vi "XOR Tester.vi"() -> ()   [LabVIEW 2013, in "Super Simple Neural Network.lvlib"]
uses:
  Super Simple Neural Network.lvlib
  <vilib>/Math Plots/3D Math Plots/3D Surface/3D Surface XCtrl/3D Surface.xctl
  <vilib>/Math Plots/3D Math Plots/3D Surface/3D Surface Datatype/3D Surface Datatype.lvclass
  Types/Stop Settings.ctl
  Types/Error Evaluation.ctl
panel:
  out "Response Surface":refnum<class "3D Plot Datatype.lvclass">[](xcontrol)
  in  "1st Hidden Layer Neurons":i32=2
  out "Goal Reached":bool=TRUE
  out "Error Trend":dbl[](graph)=[1.2002969476479681, 1.2003117160068655, 1.1995748068252734, 1.1986266775824506, 1.1980759314790428, 1.1979331980453334, 1.1976182630837475, 1.1975531304739626, 1.1975550658555898, 1.1979172951382462, 1.1980082841901254, 1.1978288179593928, 1.1976548206695512, 1.1975294735041757, 1.1971542016928627, 1.1967580661942594, 1.196216870199815, 1.195587636803456, 1.1947866780682184, 1.1937807789025867, 1.1926114580938205, 1.1911927459665133, 1.189611032453872, 1.1879425541706663, 1.1845149684498697, 1.1790670045354323, 1.17271337283506, 1.1648553404478168, 1.154971369668143, 1.1429811791798623, 1.1413485366821972, 1.1363483063148954, 1.1285959137026458, 1.1183842954352032, 1.1000568961697912, 1.083998923386862, 1.0794867997140547, 1.0684617721747578, 1.0553434826869061, 1.0396958392495204, 1.02101123534143, 0.9870568895525247, 0.9538717523120656, 0.9292072809802745, 0.9277611383844048, 0.920217692956792, 0.9084926670755543, 0.8774111592803272, 0.8469460769163291, 0.8376337144337398, 0.8100956788583408, 0.7808588146654515, 0.7464611009002428, 0.7164446834205364, 0.6860931635965195, 0.6642874827461767, 0.6461698055293237, 0.6016389331387895, 0.5521940551327592, 0.4989840147890163, 0.46441855327952186, 0.41729315960747854, 0.3703383060113925, 0.3405465537992886, 0.3273094582704069, 0.3337348036757197, 0.33928987259102134, 0.3351085676703055, 0.33232405100150914, 0.3149530937747707, 0.29789405799141794, 0.28600474402962706, 0.28456326623217576, 0.2907819179767071, 0.2921232072153035, 0.2940047293155137, 0.2879779909912136, 0.28246444258404346, 0.2756352726767302, 0.26772935920574203, 0.25842195851389893, 0.2474992301012963, 0.2273583014029358, 0.2087320931456691, 0.18863310369744024, 0.1775969638076887, 0.1592192620834864, 0.1377098111297188, 0.11267838671254482, 0.08249869363894832]
  in  "Output Neurons/Outputs":i32=1
  in  "# Inputs":i32=2
  # "The succes rate for finding \na solution to the XOR \nproblem is smaller \nthan 100%. Sometimes you \nneed to re-run\nthe example multiple times.\n\nThe values of XOR are not 0\nand 1 to present the ability\nto scale inputs and outputs\ninside the API."
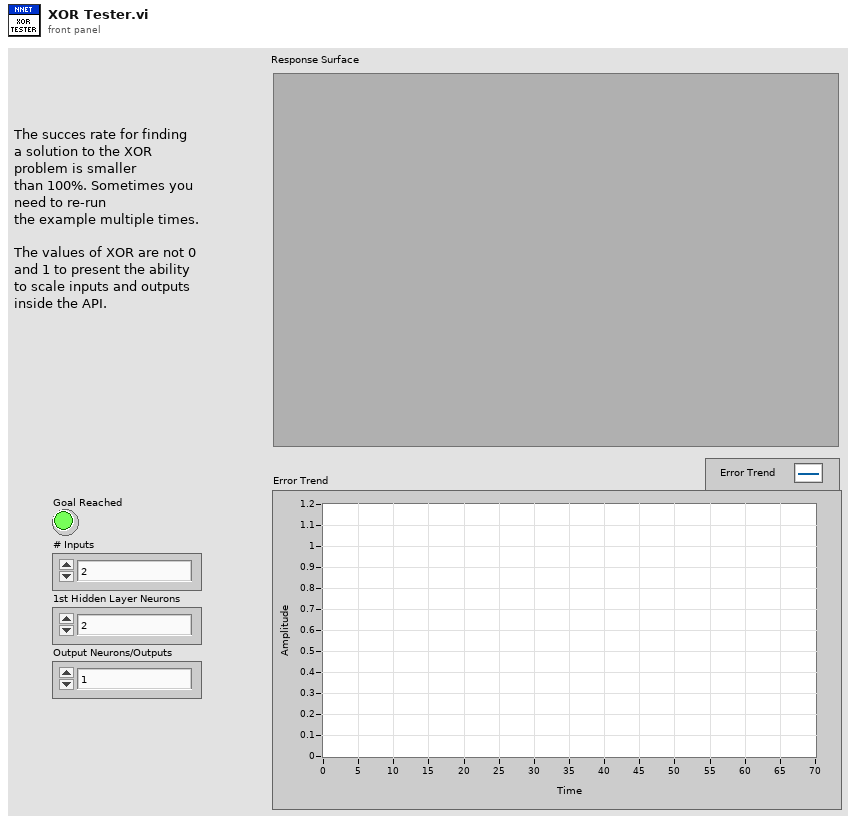
[diagram p1: front panel]
types:
  T1 = typedef "Super Simple Neural Network.lvlib/Stop Settings.ctl" = cluster{"Max Epocs":u64, "Error Goal":dbl, "Max Time (s)":dbl, "Error Evaluation":T2}
  T2 = typedef "Super Simple Neural Network.lvlib/Error Evaluation.ctl" = enum16{"Over Both Sets", "Over Validation Set", "Over Teaching Set"}
  T3 = typedef "Super Simple Neural Network.lvlib/Neural Network.ctl" = cluster{"Weigths":T4[], "Last Layer Linear":bool, "Add Bias Inputs":bool, "# Inputs":u32, "# Output Neurons/Outputs":u32, "Inputs Scaling":T5, "Outputs Scaling":T5}
  T4 = typedef "Super Simple Neural Network.lvlib/2D Array.ctl" = cluster{"2D Array":dbl[][]}
  T5 = typedef "Super Simple Neural Network.lvlib/Scaling Info.ctl" = cluster{"X Scaling Vector":dbl[], "Y Scaling Vector":dbl[]}
  T6 = typedef "Super Simple Neural Network.lvlib/Teaching Vector.ctl" = cluster{"Inputs":T7, "Expected Outputs":T7}
  T7 = typedef "Super Simple Neural Network.lvlib/1D Array.ctl" = cluster{"1D Array":dbl[]}
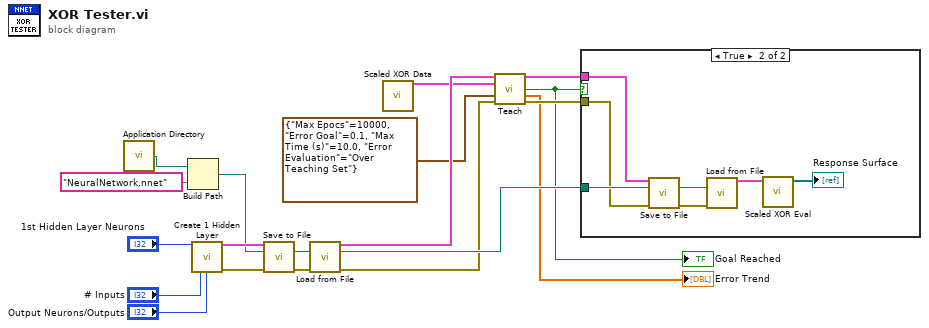
[diagram p0: block diagram]
diagram:
  n1 = call <vilib>:"Application Directory.vi"() -> ("Application Directory"=w4:path)
  n2 = Build Path(base path=w4, name or relative path="NeuralNetwork.nnet") -> (appended path=w2:path)
  n3 = call "Create 1 Hidden Layer.vi"("1st Hidden Layer Neurons"="1st Hidden Layer Neurons", "# Inputs"="# Inputs", "Output Neurons/Outputs"="Output Neurons/Outputs") -> ("Neural Network Out"=w17:T3, "Error Out"=w16:errorcluster)  [unwired: 11 in]
  n4 = call "Save to File.vi"("Neural Network In"=w17, "File Path (dialog)"=w2, "Error In"=w16) -> ("Path Used"=w1:path, "Error Out"=w19:errorcluster)  [unwired: 10 in, 1 out]
  n5 = call "Load from File.vi"("File Path (dialog)"=w1, "Error In"=w19) -> ("Neural Network Out"=w12:T3, "Used Path"=w18:path, "Error Out"=w10:errorcluster)  [unwired: 10 in, 1 out]
  n6 = call "Scaled XOR Data.vi"() -> ("XOR"=w11:T6[])  [unwired: 15 in]
  n7 = call "Teach.vi"("Neural Network In"=w12, "Teaching Set In"=w11, "Termination Settings In"=T1 {"Max Epocs"=10000, "Error Goal"=0.1, "Max Time (s)"=10.0, "Error Evaluation"=enum."Over Teaching Set"} ("Termination Settings"), "Error In"=w10) -> ("Neural Network Out"=w6:T3, "Solution Found"=w7:bool, "Error Trend Out"=→"Error Trend":dbl[], "Error Out"=w9:errorcluster)  [unwired: 8 in]
  "Goal Reached" <- w7
  n8 = case shown="True" w7 {
    tunnel: w18 -> [_ w24]
    tunnel: w6 -> [_ w23]
    tunnel: w9 -> [_ w22]
    frame False {
    }
    frame True {
      n9 = call "Save to File.vi"("Neural Network In"=w23, "File Path (dialog)"=w24, "Error In"=w22) -> ("Path Used"=w26:path, "Error Out"=w25:errorcluster)  [unwired: 10 in, 1 out]
      n10 = call "Load from File.vi"("File Path (dialog)"=w26, "Error In"=w25) -> ("Neural Network Out"=w20:T3)  [unwired: 10 in, 3 out]
      n11 = call "Scaled XOR Eval.vi"("Neural Network Out"=w20) -> ("3D Plot lvclass Array out"=→"Response Surface":refnum<class "3D Plot Datatype.lvclass">[])  [unwired: 10 in]
    }
  }
